vi "Player Info.vi"(11 "Spawn in":refnum<class "Spawn.lvclass">) -> (1 "Victory Speech":string, 2 "Name":string, 3 "Spawn out":refnum<class "Spawn.lvclass">)   [LabVIEW 2015, in "Spawn.lvclass"]
uses:
  Spawn.lvclass
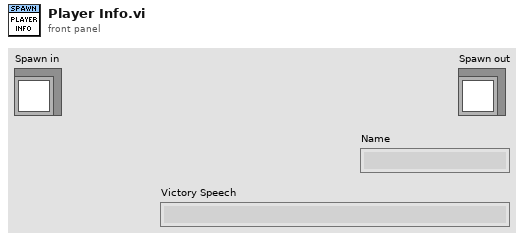
[diagram p1: front panel]
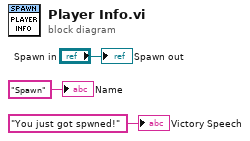
[diagram p0: block diagram]
diagram:
  "Spawn out" <- "Spawn in"
  "Name" <- "Spawn" ("Name")
  "Victory Speech" <- "You just got spwned!" ("Victory Speech")
